vi "Manual_Shooter.vi"(10 "Intake":dbl=1.0, 11 "Shooter RPM":dbl=3000.0) -> ()   [LabVIEW 2015]
uses:
  Robot Global Data.vi
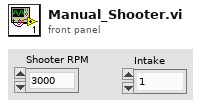
[diagram p1: front panel]
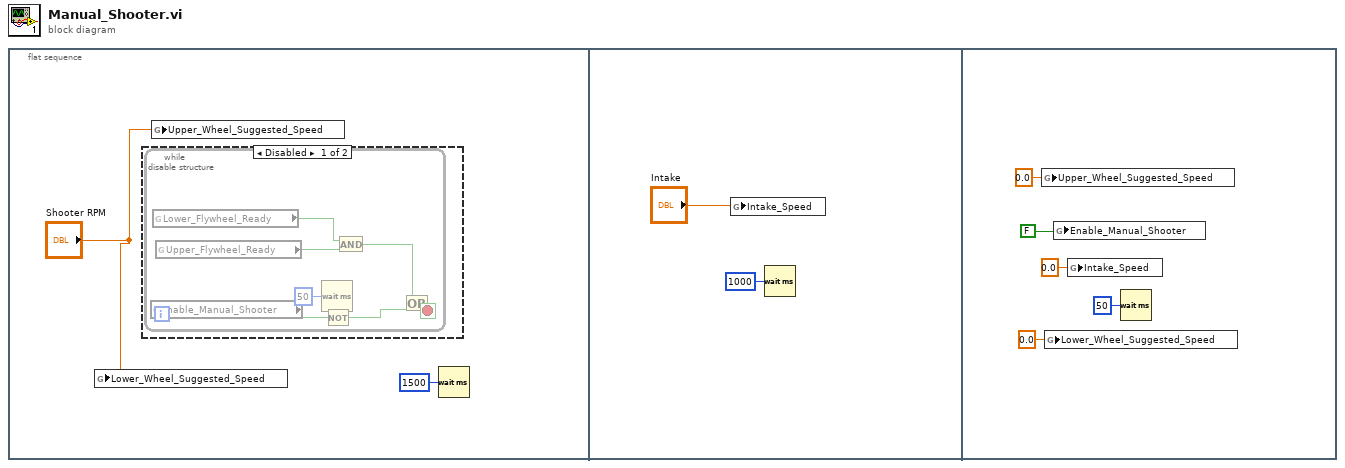
[diagram p0: block diagram]
diagram:
  n1 = flat-sequence {
    frame #0 {
      n2 = global write "Robot Global Data.vi" "Lower_Wheel_Suggested_Speed"("Shooter RPM") -> ()
      n3 = disable-structure shown="Disabled" {
        frame Disabled {
          n4 = while {
            stop <- w5 stop-if-true
            n5 = global read "Robot Global Data.vi" "Enable_Manual_Shooter"() -> (w4:bool)
            n6 = global read "Robot Global Data.vi" "Lower_Flywheel_Ready"() -> (w8:bool)
            n7 = global read "Robot Global Data.vi" "Upper_Flywheel_Ready"() -> (w9:bool)
            n8 = Wait (ms)(milliseconds to wait=u32 50) -> ()  [unwired: 1 out]
            n9 = Not(x=w4) -> (.not. x?=w3:bool)
            n10 = And(x=w8, y=w9) -> (x .and. y?=w7:bool)
            n11 = Or(x=w7, y=w3) -> (x .or. y?=w5:bool)
          }
        }
        frame Enabled {
        }
      }
      n12 = global write "Robot Global Data.vi" "Upper_Wheel_Suggested_Speed"("Shooter RPM") -> ()
      n13 = Wait (ms)(milliseconds to wait=u32 1500) -> ()  [unwired: 1 out]
    }
    frame #1 {
      n14 = global write "Robot Global Data.vi" "Intake_Speed"("Intake") -> ()
      n15 = Wait (ms)(milliseconds to wait=u32 1000) -> ()  [unwired: 1 out]
    }
    frame #2 {
      n16 = global write "Robot Global Data.vi" "Upper_Wheel_Suggested_Speed"(0.0 ("Upper_Wheel_Suggested_Speed")) -> ()
      n17 = global write "Robot Global Data.vi" "Lower_Wheel_Suggested_Speed"(0.0 ("Lower_Wheel_Suggested_Speed")) -> ()
      n18 = global write "Robot Global Data.vi" "Enable_Manual_Shooter"(FALSE ("Enable_Shooter")) -> ()
      n19 = global write "Robot Global Data.vi" "Intake_Speed"(0.0 ("Intake_Speed")) -> ()
      n20 = Wait (ms)(milliseconds to wait=u32 50) -> ()  [unwired: 1 out]
    }
  }
